vi "ROI_FromFirstFrame_version2.vi"(8 "error in":errorcluster, 11 "QSM_ShiftRegister_TEST in":T1 {"ROI Process"."Particle Variables" items=["Center of Mass X", "Center of Mass Y", "First Pixel X", "First Pixel Y", "Bounding Rect Left", "Bounding Rect Top", "Bounding Rect Right", "Bounding Rect Bottom", "Max Feret Diameter Start X", "Max Feret Diameter Start Y", "Max Feret Diameter End X", "Max Feret Diameter End Y", "Max Horiz. Segment Length Left", "Max Horiz. Segment Length Right", "Max Horiz. Segment Length Row", "-", "Bounding Rect Width", "Bounding Rect Height", "Bounding Rect Diagonal", "Perimeter", "Convex Hull Perimeter", "Holes' Perimeter", "Max Feret Diameter", "Equivalent Ellipse Major Axis", "Equivalent Ellipse Minor Axis", "Equivalent Ellipse Minor Axis (Feret)", "Equivalent Rect Long Side", "Equivalent Rect Short Side", "Equivalent Rect Diagonal", "Equivalent Rect Short Side (Feret)", "Average Horiz. Segment Length", "Average Vert. Segment Length", "Hydraulic Radius", "Waddel Disk Diameter", "-", "Area", "Holes' Area", "Particle & Holes' Area", "Convex Hull Area", "Image Area", "-", "Number of Holes", "Number of Horiz. Segments", "Number of Vert. Segments", "-", "Orientation", "Max Feret Diameter Orientation", "-", "% Area/Image Area", "% Area/(Particle & Holes' Area)", "Ratio of Equivalent Ellipse Axes", "Ratio of Equivalent Rect Sides", "-", "Elongation Factor", "Compactness Factor", "Heywood Circularity Factor", "Type Factor", "-", "Sum X", "Sum Y", "Sum XX", "Sum XY", "Sum YY", "Sum XXX", "Sum XXY", "Sum XYY", "Sum YYY", "-", "Moment of Inertia XX", "Moment of Inertia XY", "Moment of Inertia YY", "Moment of Inertia XXX", "Moment of Inertia XXY", "Moment of Inertia XYY", "Moment of Inertia YYY", "Norm. Moment of Inertia XX", "Norm. Moment of Inertia XY", "Norm. Moment of Inertia YY", "Norm. Moment of Inertia XXX", "Norm. Moment of Inertia XXY", "Norm. Moment of Inertia XYY", "Norm. Moment of Inertia YYY", "Hu Moment 1", "Hu Moment 2", "Hu Moment 3", "Hu Moment 4", "Hu Moment 5", "Hu Moment 6", "Hu Moment 7"]; "ROI Process"."Particle Measurements (Pixels)" format="%.2f"; "ROI Process"."ROIS"."Contours"."Type" items=["No Selection", "Point", "Line", "Rectangle", "Oval", "Polygon", "Freehand Region", "Annulus", "Unused2", "Unused3", "Broken Line", "Freehand Line", "Rotated Rectangle"]; "Single Image Results"."ROI Results"."LIMLOCALMETADATA"."dTimeMSec" format="%.2f"}) -> (0 "error out":errorcluster, 1 "Original Image (I16)":T8, 2 "ROI Out (U8)":T8(plugin-control), 3 "QSM_ShiftRegister_TEST out":T1 {"ROI Process"."Particle Variables" items=["Center of Mass X", "Center of Mass Y", "First Pixel X", "First Pixel Y", "Bounding Rect Left", "Bounding Rect Top", "Bounding Rect Right", "Bounding Rect Bottom", "Max Feret Diameter Start X", "Max Feret Diameter Start Y", "Max Feret Diameter End X", "Max Feret Diameter End Y", "Max Horiz. Segment Length Left", "Max Horiz. Segment Length Right", "Max Horiz. Segment Length Row", "-", "Bounding Rect Width", "Bounding Rect Height", "Bounding Rect Diagonal", "Perimeter", "Convex Hull Perimeter", "Holes' Perimeter", "Max Feret Diameter", "Equivalent Ellipse Major Axis", "Equivalent Ellipse Minor Axis", "Equivalent Ellipse Minor Axis (Feret)", "Equivalent Rect Long Side", "Equivalent Rect Short Side", "Equivalent Rect Diagonal", "Equivalent Rect Short Side (Feret)", "Average Horiz. Segment Length", "Average Vert. Segment Length", "Hydraulic Radius", "Waddel Disk Diameter", "-", "Area", "Holes' Area", "Particle & Holes' Area", "Convex Hull Area", "Image Area", "-", "Number of Holes", "Number of Horiz. Segments", "Number of Vert. Segments", "-", "Orientation", "Max Feret Diameter Orientation", "-", "% Area/Image Area", "% Area/(Particle & Holes' Area)", "Ratio of Equivalent Ellipse Axes", "Ratio of Equivalent Rect Sides", "-", "Elongation Factor", "Compactness Factor", "Heywood Circularity Factor", "Type Factor", "-", "Sum X", "Sum Y", "Sum XX", "Sum XY", "Sum YY", "Sum XXX", "Sum XXY", "Sum XYY", "Sum YYY", "-", "Moment of Inertia XX", "Moment of Inertia XY", "Moment of Inertia YY", "Moment of Inertia XXX", "Moment of Inertia XXY", "Moment of Inertia XYY", "Moment of Inertia YYY", "Norm. Moment of Inertia XX", "Norm. Moment of Inertia XY", "Norm. Moment of Inertia YY", "Norm. Moment of Inertia XXX", "Norm. Moment of Inertia XXY", "Norm. Moment of Inertia XYY", "Norm. Moment of Inertia YYY", "Hu Moment 1", "Hu Moment 2", "Hu Moment 3", "Hu Moment 4", "Hu Moment 5", "Hu Moment 6", "Hu Moment 7"]; "ROI Process"."Particle Measurements (Pixels)" format="%.2f"; "ROI Process"."ROIS"."Contours"."Type" items=["No Selection", "Point", "Line", "Rectangle", "Oval", "Polygon", "Freehand Region", "Annulus", "Unused2", "Unused3", "Broken Line", "Freehand Line", "Rotated Rectangle"]; "Single Image Results"."ROI Results"."LIMLOCALMETADATA"."dTimeMSec" format="%.2f"}, 4 "LIMLOCALMETADATA":T6 {"dTimeMSec" format="%.2f"})   [LabVIEW 2014]
uses:
  <vilib>/vision/Image Controls.llb/IMAQ Image.ctl
  ND2_Reader_32bit/controls/cluster_LIMLOCALMETADATA.ctl
  QSM/Queue_TEST/Controls/QSM_ShiftRegister.ctl
  QSM/QueueMaintenance/TypeDef/QSMRef_ALL.ctl
  QSM/Queue_TESTGUIUPDATE/Controls/QSM_Reference.ctl
  QSM/Queue_TESTGUIUPDATE/Controls/QSM_DataType.ctl
  QSM/Queue_TESTGUIUPDATE/Controls/QSM_RunStates.ctl
  QSM/Queue_TEST/Controls/QSM_Reference.ctl
  QSM/Queue_TEST/Controls/QSM_DataType.ctl
  QSM/Queue_TEST/Controls/QSM_RunStates.ctl
  Custom Controls/cluster - Image Results.ctl
  ND2_Reader_32bit/ND2_Reader_32.lvlib
  QSM/Queue_TESTGUIUPDATE/GUIUpdateQSM.lvlib
  QSM/Queue_TEST/TestQSM.lvlib
  QSM/QueueMaintenance/QueueMaintenance.lvlib
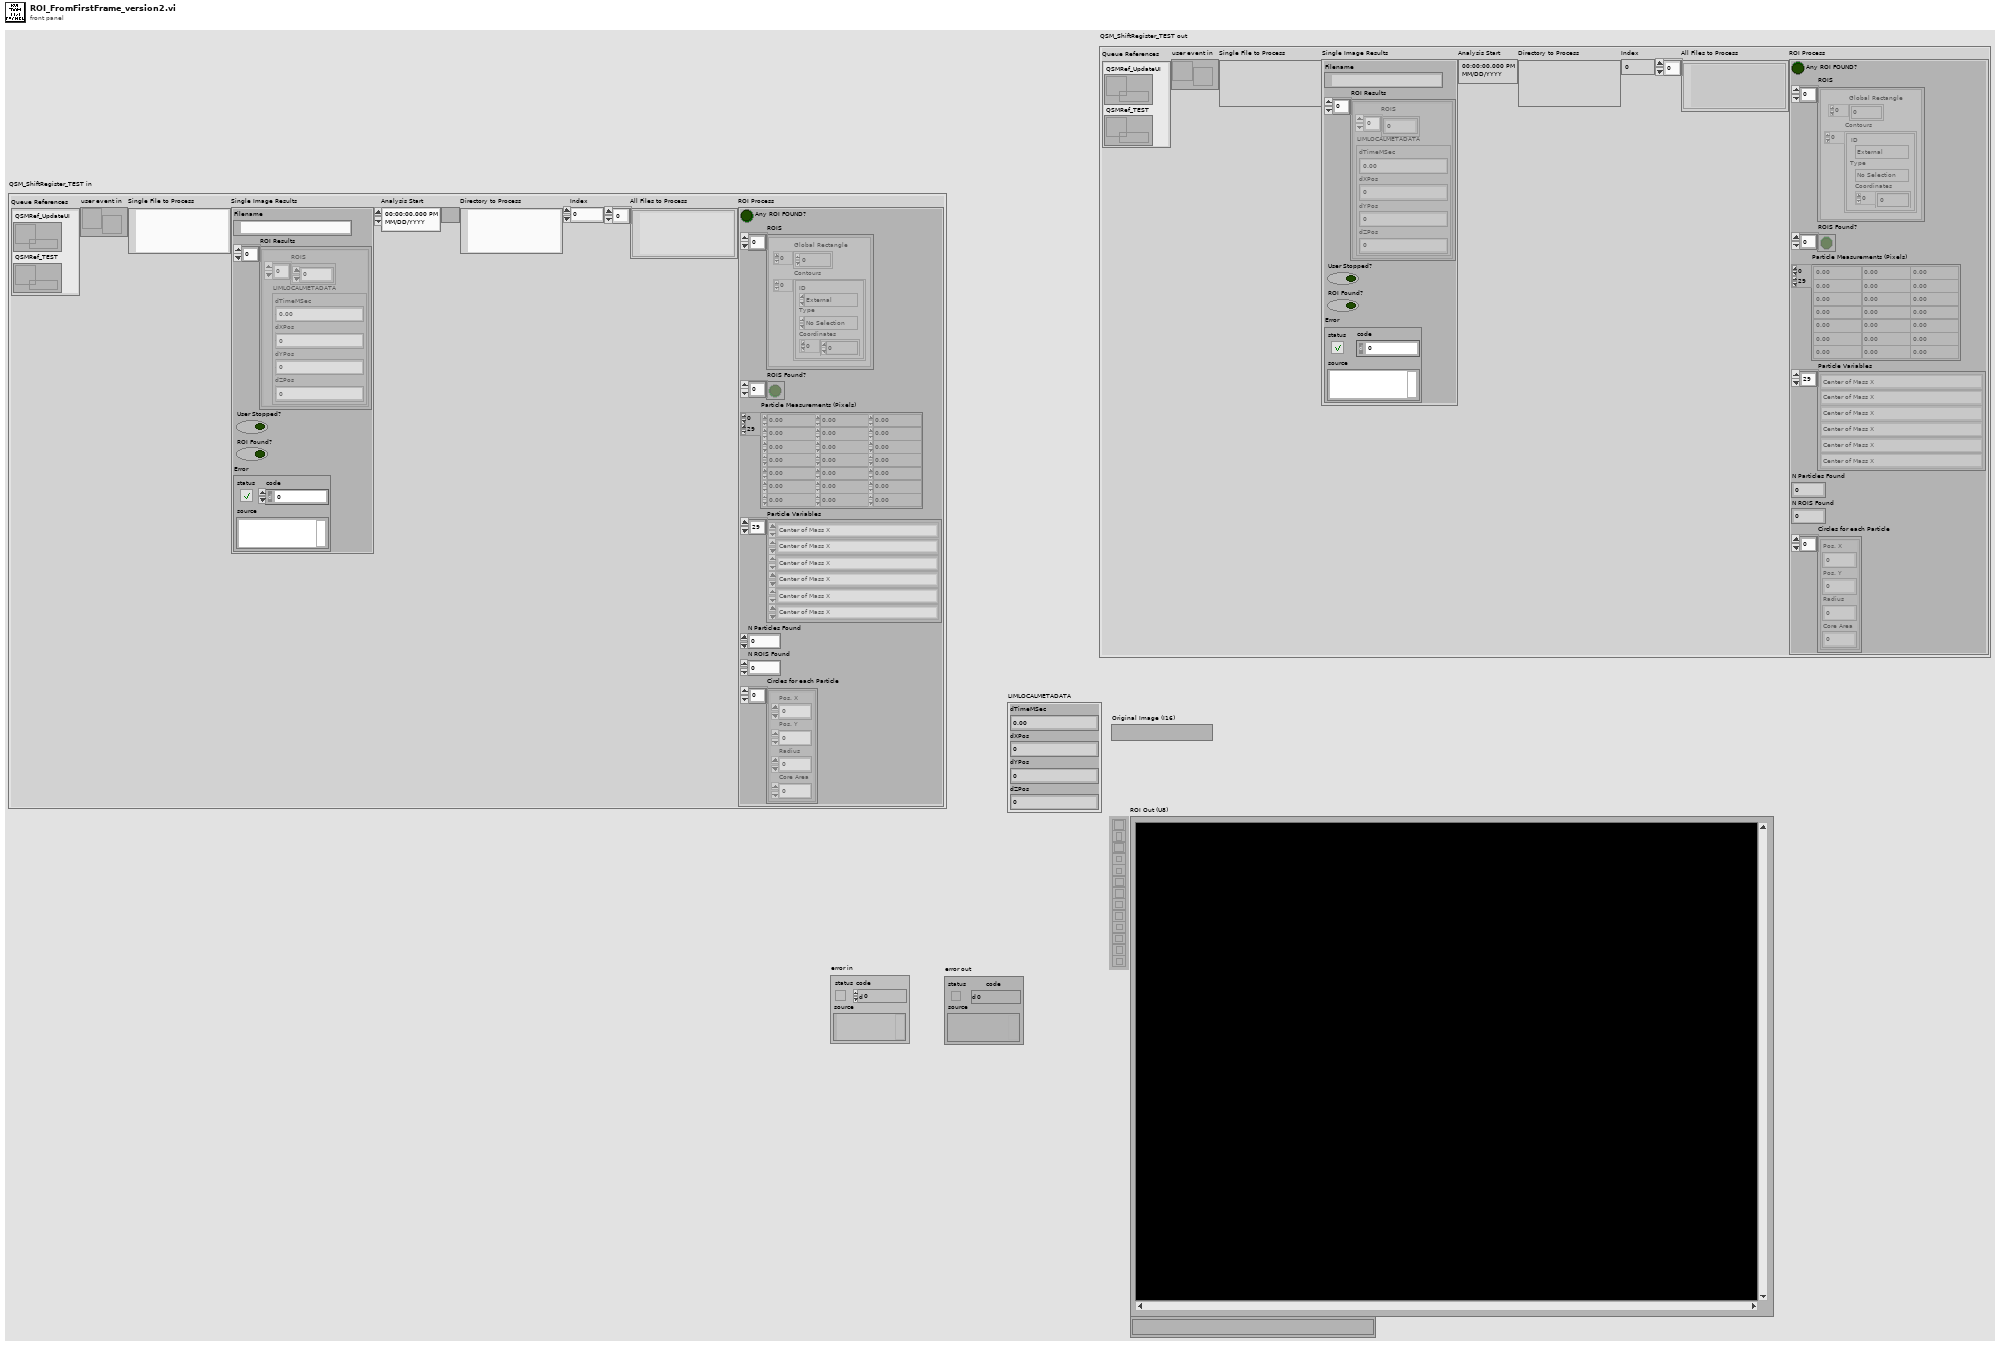
[diagram p1: front panel]
types:
  T1 = typedef "TestQSM.lvlib/QSM_ShiftRegister.ctl" = cluster{"Queue References":T2, "user event in":refnum<user-event>, "Single File to Process":path, "Single Image Results":T5, "Analysis Start":timestamp, "Directory to Process":path, "Index":i32, "All Files to Process":path[], "ROI Process":cluster{"Any ROI FOUND?":bool, "ROIS":T7[], "ROIS Found?":bool[], "Particle Measurements (Pixels)":dbl[][], "Particle Variables":i32[], "N Particles Found":i32, "N ROIS Found":i32, "Circles for each Particle":cluster{"Pos. X":i32, "Pos. Y":i32, "Radius":i32, "Core Area":i32}[]}}
  T2 = typedef "QueueMaintenance.lvlib/QSMRef_ALL.ctl" = cluster{"QSMRef_UpdateUI":T3, "QSMRef_TEST":T4}
  T3 = typedef "GUIUpdateQSM.lvlib/QSM_Reference.ctl" = refnum<queue>
  T4 = typedef "TestQSM.lvlib/QSM_Reference.ctl" = refnum<queue>
  T5 = typedef "cluster - Image Results.ctl" = cluster{"Filename":path, "ROI Results":cluster{"ROIS":dbl[], "LIMLOCALMETADATA":T6}[], "User Stopped?":bool, "ROI Found?":bool, "Error":errorcluster}
  T6 = typedef "cluster_LIMLOCALMETADATA.ctl" = cluster{"dTimeMSec":dbl, "dXPos":dbl, "dYPos":dbl, "dZPos":dbl}
  T7 = typedef "ROI Descriptor" = cluster{"Global Rectangle":i32[], "Contours":cluster{"ID":enum32{"External", "Internal"}, "Type":u32, "Coordinates":i32[]}[]}
  T8 = typedef "IMAQ Image.ctl" = refnum<image>
  T9 = typedef "Image Type" = u32
  T10 = cluster{"Pos. X":i32, "Pos. Y":i32, "Radius":i32, "Core Area":i32}[]
  T11 = cluster{"Pos. X":i32, "Pos. Y":i32, "Radius":i32, "Core Area":i32}
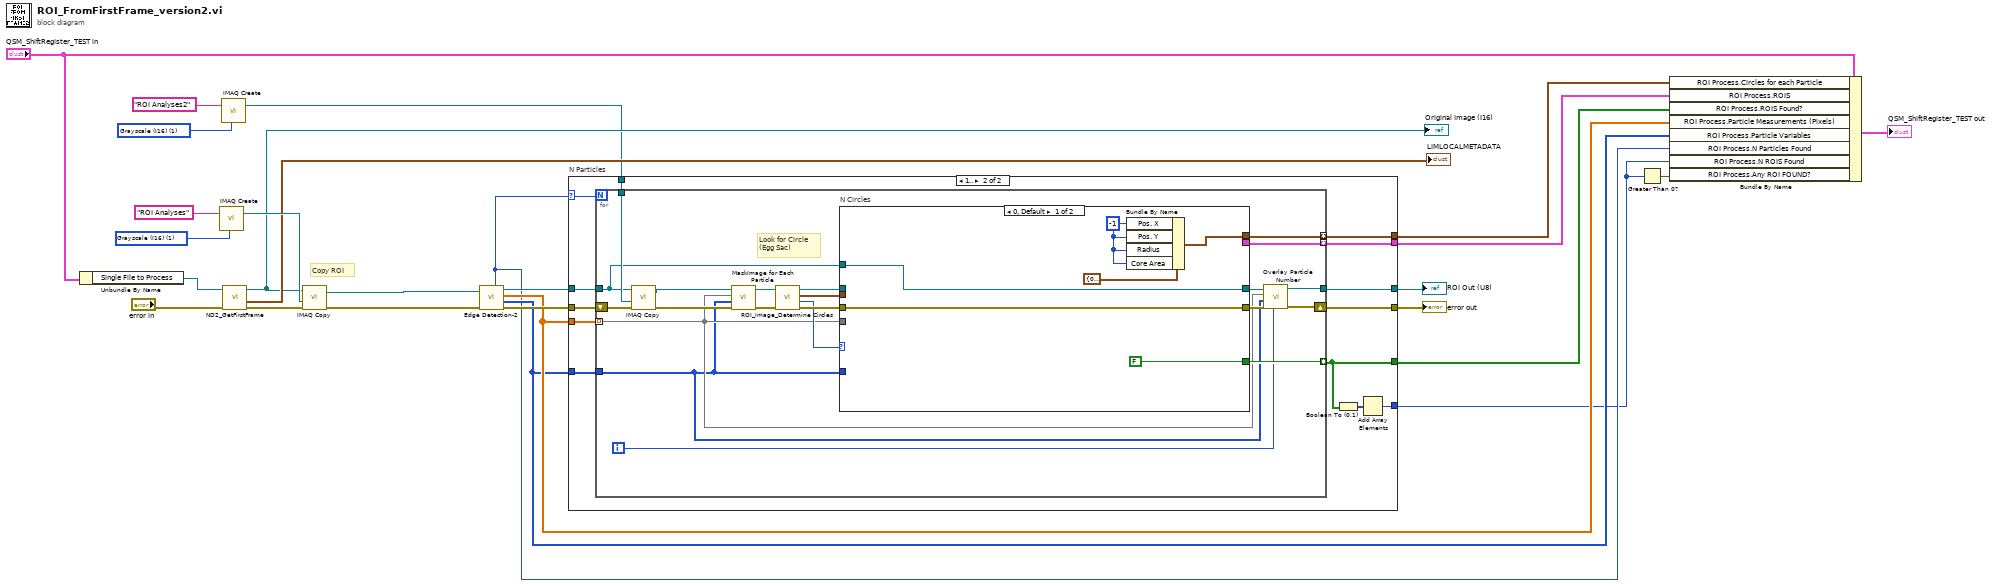
[diagram p0: block diagram]
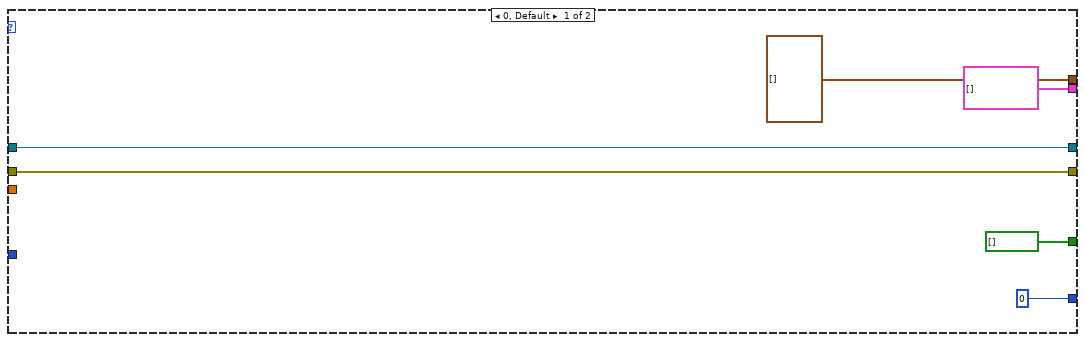
[diagram p2: hidden frame]
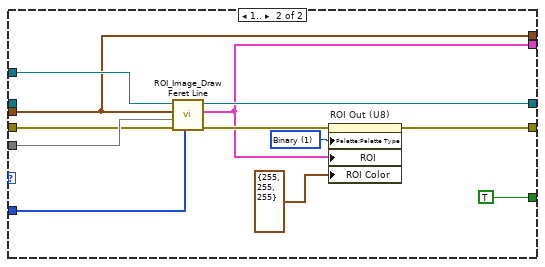
[diagram p3: hidden frame]
diagram:
  w14 = T9 1 items=["Grayscale (U8)", "Grayscale (I16)", "Grayscale (SGL)", "Complex (CSG)", "RGB (U32)", "HSL (U32)", "RGB (U64)", "Grayscale (U16)"] ("Image Type")
  w23 = T9 1 items=["Grayscale (U8)", "Grayscale (I16)", "Grayscale (SGL)", "Complex (CSG)", "RGB (U32)", "HSL (U32)", "RGB (U64)", "Grayscale (U16)"] ("Image Type")
  # "Copy ROI"
  n1 = Unbundle By Name("QSM_ShiftRegister_TEST in") -> ("Single File to Process"=w11:path)
  n2 = call "IMAQ Create"("Image Name"="ROI Analyses", "Image Type"=w23) -> ("New Image"=w21:T8)  [unwired: 3 in, 1 out]
  n3 = call "IMAQ Create"("Image Name"="ROI Analyses2", "Image Type"=w14) -> ("New Image"=w12:T8)  [unwired: 3 in, 1 out]
  n4 = call "ND2_GetFirstFrame.vi"("error in (no error)"="error in", "FilePath"=w11) -> ("error out"=w22:errorcluster, "LIMLOCALMETADATA"=→"LIMLOCALMETADATA":T6, "Image out"=w19:T8)  [unwired: 7 in]
  "Original Image (I16)" <- w19
  n5 = call "IMAQ Copy"("error in (no error)"=w22, "Image Dst"=w21, "Image Src"=w19) -> ("error out"=w15:errorcluster, "Image Dst Out"=w16:T8)  [unwired: 3 in]
  n6 = call "Edge Detection-2.vi"("error in"=w15, "Image"=w16) -> ("error out"=w17:errorcluster, "Particle Variables"=w5:i32[], "Particle Measurements (Pixels)"=w6:dbl[][], "Image Out"=w18:T8, "Number of Particles"=w4:i32)  [unwired: 5 in]
  n7 = case "N Particles" shown="1.." w4 {
    selector: w4 -> [_ w39]
    tunnel: [w32 w46] -> w27
    tunnel: [w33 w45] -> w25
    tunnel: w6 -> [_ w44]
    tunnel: w5 -> [_ w43]
    tunnel: [T7[] [] w42] -> w8
    tunnel: w18 -> [w33 w41]
    tunnel: w17 -> [w32 w40]
    tunnel: [bool[] [] w37] -> w7
    tunnel: w12 -> [_ w38]
    tunnel: [0 w36] -> w3
    tunnel: [T10 [] w34] -> w1
    frame 0, Default {
    }
    frame 1.. {
      n8 = for {
        N: w39 -> [_]
        tunnel: [w50] -> w45
        tunnel: w44 -> [w52] mode=indexing
        tunnel: w43 -> [w51]
        tunnel: [w66] -> w42 mode=indexing
        tunnel: w41 -> [w55]
        tunnel: [w62] -> w37 mode=indexing
        shift-right: [w49] -> w46
        shift-left: w40 -> [w59]
        tunnel: w38 -> [w56]
        tunnel: [w47] -> w34 mode=indexing
        i -> [w48]
        # "Look for Circle\n(Egg Sac)"
        n9 = call "IMAQ Copy"("error in (no error)"=w59, "Image Dst"=w56, "Image Src"=w55) -> ("error out"=w57:errorcluster, "Image Dst Out"=w58:T8)  [unwired: 3 in]
        n10 = call "MaskImage for Each Particle.vi"("error in"=w57, "Particle Variables"=w51, "Particle Measurements (Pixels)"=w52, "Image"=w58) -> ("error out"=w60:errorcluster, "Image Out"=w61:T8)  [unwired: 6 in]
        n11 = call "ROI_Image_Determine Circles.vi"("error in (no error)"=w60, "Image in"=w61) -> ("error out"=w67:errorcluster, "N Circles"=w63:i32, "Biggest Circles Data"=w64:T11, "Image out"=w65:T8)  [unwired: 6 in]
        n12 = case "N Circles" shown="0, Default" w63 {
          tunnel: [w73 w84] -> w53
          tunnel: [w71 w83] -> w54
          tunnel: w52 -> [_ w81]
          tunnel: w51 -> [_ w80]
          tunnel: w67 -> [w73 w79]
          tunnel: [_ w78] -> w66
          tunnel: w65 -> [_ _]
          tunnel: w64 -> [_ w74]
          tunnel: [FALSE TRUE] -> w62
          tunnel: w55 -> [w71 w75]
          tunnel: [w69 w74] -> w47
          frame 0, Default {
            w68 = -1 ("Pos. X")
            n13 = Bundle By Name(cluster=T11 {"Pos. X"=0, "Pos. Y"=0, "Radius"=0, "Core Area"=0} ("Circles Data"), "Pos. X"=w68, "Pos. Y"=w68, "Radius"=w68, "Core Area"=w68) -> (w69:T11)
          }
          frame 1.. {
            w85 = u32 1 items=["Grayscale", "Binary", "Gradient", "Rainbow", "Temperature", "User Defined"] ("Palette")
            n14 = call "ROI_Image_Draw Feret Line.vi"("Pixel Measurements"=w80, "error in (no error)"=w79, "Particle Measurements (Pixels)"=w81, "Circle Data"=w74, "Image in"=w75) -> ("error out"=w82:errorcluster, "ROI"=w78:T7, "Image out"=w83:T8)  [unwired: 4 in]
            n15 = property on="ROI Out (U8)" class="ImageControl"(error in=w82, "Palette:Palette Type"=w85, "ROI"=w78, "ROI Color"=cluster{"Red":u8, "Green":u8, "Blue":u8} {"Red"=255, "Green"=255, "Blue"=255}) -> (error out=w84:errorcluster)  [unwired: 1 in, 1 out]
          }
        }
        n16 = call "Overlay Particle Number.vi"("Particle Index"=w48, "error in"=w53, "Particle Variables"=w51, "Particle Measurements (Pixels)"=w52, "Image"=w54) -> ("error out"=w49:errorcluster, "Image Out"=w50:T8)  [unwired: 5 in]
      }
      n17 = Boolean To (0,1)(Boolean=w37) -> (0, 1=w35:i16[])
      n18 = Add Array Elements(numeric array=w35) -> (sum=w36:i16)
    }
  }
  "error out" <- w27
  "ROI Out (U8)" <- w25
  n19 = Greater Than 0?(x=w3) -> (x > 0?=w2:bool)
  n20 = Bundle By Name(cluster="QSM_ShiftRegister_TEST in", "ROI Process.Circles for each Particle"=w1, "ROI Process.ROIS"=w8, "ROI Process.ROIS Found?"=w7, "ROI Process.Particle Measurements (Pixels)"=w6, "ROI Process.Particle Variables"=w5, "ROI Process.N Particles Found"=w4, "ROI Process.N ROIS Found"=w3, "ROI Process.Any ROI FOUND?"=w2) -> (→"QSM_ShiftRegister_TEST out":T1)
